vi "索引簇检查.vi"(4 "簇":T1, 6 "CtlRef":refnum<vi>, 7 "范围":bool, 8 "错误输入（无错误）":errorcluster, 11 "queue out":refnum<queue>) -> (0 "错误输出":errorcluster)   [LabVIEW 2021]
uses:
  LabView Lib/QueueLib/QueueLib.lvlib
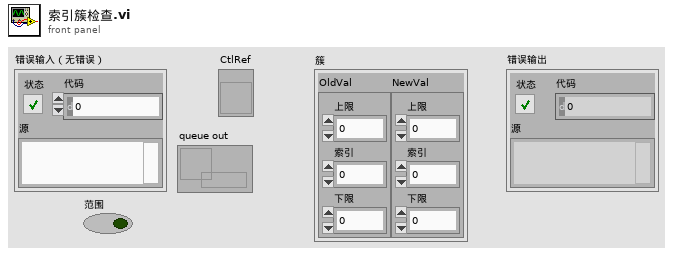
[diagram p1: front panel]
types:
  T1 = cluster{"OldVal":cluster{"上限":u32, "索引":i32, "下限":u32}, "NewVal":cluster{"上限":u32, "索引":i32, "下限":u32}}
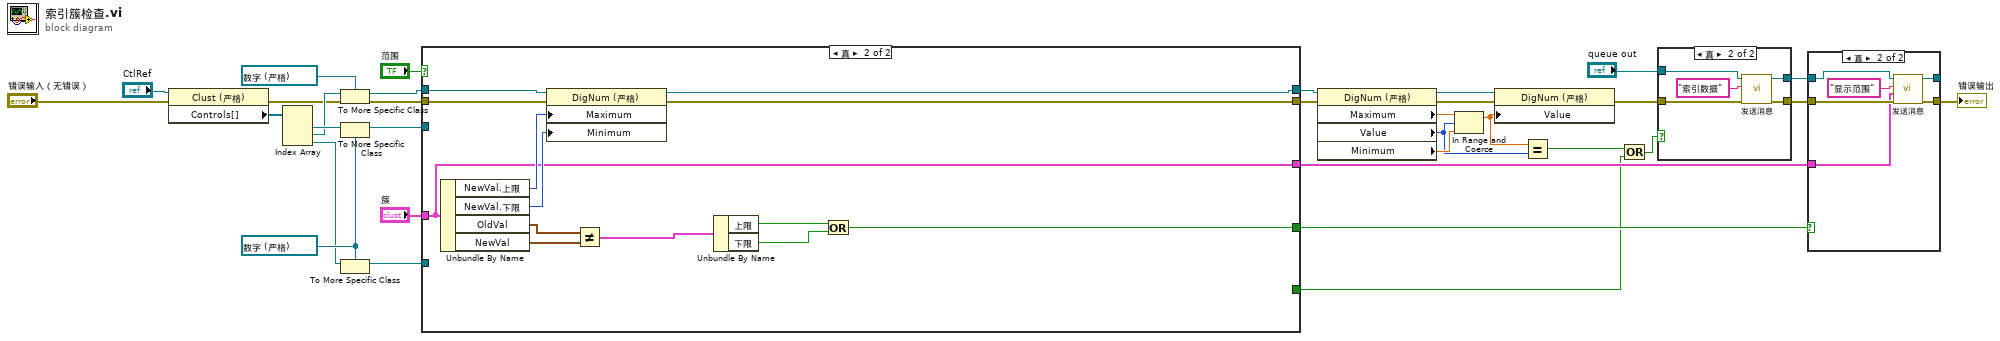
[diagram p0: block diagram]
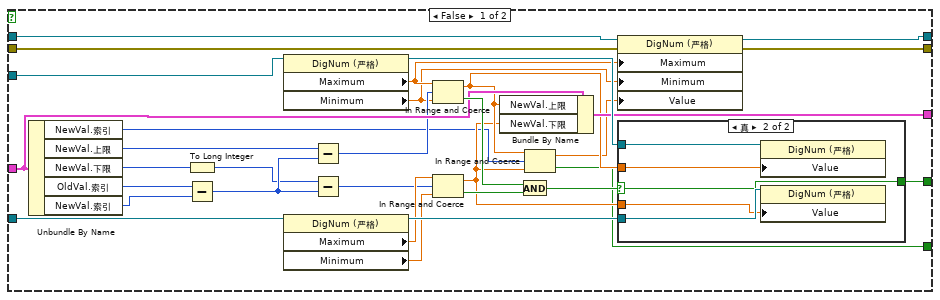
[diagram p4: hidden frame]
diagram:
  w19 = refnum<vi> refnum ("上限")
  n1 = property class="Clust (严格)"(reference="CtlRef", error in="错误输入（无错误）") -> (error out=w4:errorcluster, "Controls[]"=w31:refnum<vi>[])  [unwired: 1 out]
  n2 = Index Array(array=w31) -> (element #1=w32:refnum<vi>, element #2=w22:refnum<vi>, element #3=w18:refnum<vi>)  [unwired: 3 in]
  n3 = To More Specific Class(target class=refnum<vi> refnum ("索引"), reference=w22, error in=w4) -> (specific class reference=w21:refnum<vi>, error out=w5:errorcluster)
  n4 = To More Specific Class(target class=w19, reference=w32) -> (specific class reference=w12:refnum<vi>)  [unwired: 1 in, 1 out]
  n5 = To More Specific Class(target class=w19, reference=w18) -> (specific class reference=w13:refnum<vi>)  [unwired: 1 in, 1 out]
  n6 = case shown="真" "范围" {
    tunnel: w5 -> [w40 w83]
    tunnel: [w39 w82] -> w28
    tunnel: "簇" -> [w52 w74]
    tunnel: w21 -> [w64 w79]
    tunnel: [w41 w78] -> w17
    tunnel: w13 -> [w63 _]
    tunnel: w12 -> [w62 _]
    tunnel: [w56 w72] -> w8
    tunnel: [w55 w74] -> w7
    tunnel: [w37 _] -> w2
    frame False {
      n7 = Unbundle By Name(w52) -> ("NewVal.索引"=w42:i32, "NewVal.上限"=w46:u32, "NewVal.下限"=w49:u32, "OldVal.索引"=w51:i32, "NewVal.索引"=w50:i32)
      n8 = To Long Integer(number=w49) -> (32bit integer=w36:i32)
      n9 = Subtract(x=w51, y=w50) -> (x-y=w47:i32)
      n10 = property class="DigNum (严格)"(reference=w62) -> (reference out=w61:refnum<vi>, "Maximum"=w35:dbl, "Minimum"=w34:dbl)  [unwired: 1 in, 1 out]
      n11 = property class="DigNum (严格)"(reference=w63) -> (reference out=w60:refnum<vi>, "Maximum"=w54:dbl, "Minimum"=w53:dbl)  [unwired: 1 in, 1 out]
      n12 = Subtract(x=w46, y=w47) -> (x-y=w45:u32)
      n13 = Subtract(x=w36, y=w47) -> (x-y=w48:i32)
      n14 = In Range and Coerce(upper limit=w35, x=w45, lower limit=w34) -> (coerced(x)=w44:dbl, In Range?=w59:bool)
      n15 = In Range and Coerce(upper limit=w54, x=w48, lower limit=w53) -> (coerced(x)=w43:dbl, In Range?=w58:bool)
      n16 = Bundle By Name(cluster=w52, "NewVal.上限"=w44, "NewVal.下限"=w43) -> (w55:T1)
      n17 = And(x=w59, y=w58) -> (x .and. y?=w57:bool)
      n18 = In Range and Coerce(upper limit=w44, x=w42, lower limit=w43) -> (coerced(x)=w38:dbl, In Range?=w37:bool)
      n19 = property class="DigNum (严格)"(reference=w64, error in=w40, "Maximum"=w35, "Minimum"=w34, "Value"=w38) -> (reference out=w41:refnum<vi>, error out=w39:errorcluster)
      n20 = case shown="真" w57 {
        selector: w57 -> [w65 w66]
        tunnel: w61 -> [_ w70]
        tunnel: w44 -> [_ w68]
        tunnel: w43 -> [_ w67]
        tunnel: w60 -> [_ w69]
        tunnel: [w65 w66] -> w56
        frame False {
        }
        frame True {
          n21 = property class="DigNum (严格)"(reference=w70, "Value"=w68) -> ()  [unwired: 1 in, 2 out]
          n22 = property class="DigNum (严格)"(reference=w69, "Value"=w67) -> ()  [unwired: 1 in, 2 out]
        }
      }
    }
    frame True {
      n23 = Unbundle By Name(w74) -> ("NewVal.上限"=w81:u32, "NewVal.下限"=w80:u32, "OldVal"=w77:cluster{"上限":u32, "索引":i32, "下限":u32}, "NewVal"=w76:cluster{"上限":u32, "索引":i32, "下限":u32})
      n24 = property on="属性节点" class="DigNum (严格)"(reference=w79, error in=w83, "Maximum"=w81, "Minimum"=w80) -> (reference out=w78:refnum<vi>, error out=w82:errorcluster)
      n25 = Not Equal?(x=w77, y=w76) -> (x != y?=w75:cluster{"上限":bool, "索引":bool, "下限":bool})
      n26 = Unbundle By Name(w75) -> ("上限"=w73:bool, "下限"=w71:bool)
      n27 = Or(x=w73, y=w71) -> (x .or. y?=w72:bool)
    }
  }
  n28 = property on="属性节点" class="DigNum (严格)"(reference=w17, error in=w28) -> (reference out=w16:refnum<vi>, error out=w25:errorcluster, "Maximum"=w26:dbl, "Value"=w14:i32, "Minimum"=w27:dbl)
  n29 = In Range and Coerce(upper limit=w26, x=w14, lower limit=w27) -> (coerced(x)=w15:dbl)  [unwired: 1 out]
  n30 = property on="属性节点" class="DigNum (严格)"(reference=w16, error in=w25, "Value"=w15) -> (error out=w29:errorcluster)  [unwired: 1 out]
  n31 = Equal?(x=w15, y=w14) -> (x = y?=w1:bool)
  n32 = Or(x=w1, y=w2) -> (x .or. y?=w3:bool)
  n33 = case shown="真" w3 {
    tunnel: w29 -> [w84 w90]
    tunnel: "queue out" -> [w85 w89]
    tunnel: [w84 w88] -> w11
    tunnel: [w85 w86] -> w9
    frame False {
    }
    frame True {
      n34 = call-poly "发送消息.vi"("错误输入（无错误）"=w90, "消息"="索引数据", "输入队列"=w89) -> ("错误输出"=w88:errorcluster, "输出队列"=w86:refnum<queue>)  [unwired: 7 in]
    }
  }
  n35 = case shown="真" w8 {
    tunnel: w11 -> [w91 w98]
    tunnel: w9 -> [w92 w97]
    tunnel: [w91 w96] -> w10
    tunnel: [w92 w95] -> _
    tunnel: w7 -> [_ w94]
    frame False {
    }
    frame True {
      n36 = call-poly "发送消息.vi"("错误输入（无错误）"=w98, "数据"=w94, "消息"="显示范围", "输入队列"=w97) -> ("错误输出"=w96:errorcluster, "输出队列"=w95:refnum<queue>)  [unwired: 6 in]
    }
  }
  "错误输出" <- w10
